vi "Create Sessions - NSess.vi"(7 "serial configuration":T1, 8 "error in":errorcluster, 9 "reset":bool, 11 "session reservation in":refnum<class "Session Reservation.lvclass">) -> (0 "error out":errorcluster, 1 "channel lists":string[](array[string]), 2 "sessions":refnum<visa-resource-name>[](array[refnum]), 3 "session reservation out":refnum<class "Session Reservation.lvclass">)   [LabVIEW 2020, in "MeasurementLink 34401.lvlib"]
doc: "Create the 34401 driver sessions from the <b>session reservation in</b>."
uses:
  MeasurementLink 34401.lvlib
  <vilib>/MeasurementLink/MeasurementLink Session Management/Session Reservation/Session Reservation.lvclass
  b3cb301c-7684-4518-818f-a956a366db36.vi
  Instrument/Instrument.lvclass
  C:/Program Files/National Instruments/LabVIEW 2020/vi.lib/MeasurementLink/MeasurementLink Instrument/IInstrument/IInstrument.lvclass
  <vilib>/MeasurementLink/MeasurementLink Session Management/Session Reservation/Create Sessions Dispatcher.vi
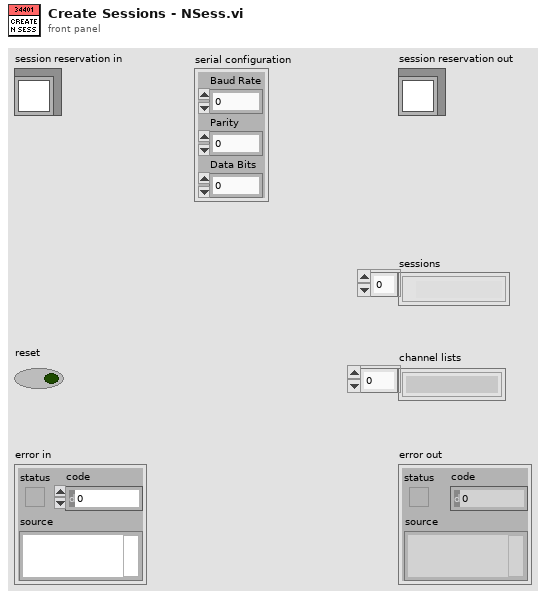
[diagram p1: front panel]
types:
  T1 = cluster{"Baud Rate":u32, "Parity":u16, "Data Bits":u16}
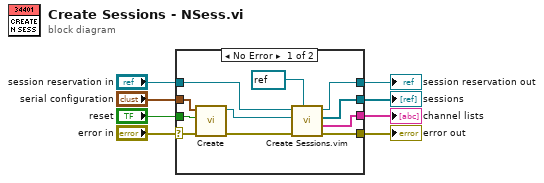
[diagram p0: block diagram]
diagram:
  n1 = case shown="No Error" "error in" {
    selector: "error in" -> [w18 w21]
    tunnel: [w13 w21] -> w7
    tunnel: [w15 w20] -> w5
    tunnel: "session reservation in" -> [w16 w20]
    tunnel: "serial configuration" -> [w19 _]
    tunnel: "reset" -> [w17 _]
    tunnel: [w12 _] -> w1
    tunnel: [w11 _] -> w3
    frame No Error {
      n2 = call "Create.vi"("error in"=w18, "reset"=w17, "serial configuration"=w19) -> ("error out"=w14:errorcluster, "instrument out"=w10:refnum<class "Instrument.lvclass">)  [unwired: 7 in]
      n3 = call "Create Sessions.vim"("session type"=refnum<visa-resource-name> refnum ("session"), "error in"=w14, "instrument"=w10, "session reservation in"=w16) -> ("error out"=w13:errorcluster, "channel lists"=w11:string[], "sessions"=w12:refnum<visa-resource-name>[], "session reservation out"=w15:refnum<class "Session Reservation.lvclass">)  [unwired: 4 in]
    }
    frame Error {
    }
  }
  "error out" <- w7
  "session reservation out" <- w5
  "channel lists" <- w3
  "sessions" <- w1
